vi "TEST_DialogValuesMatchINI.vi"() -> ()   [LabVIEW 2016]
uses:
  controls/ActiveDiffArgs.ctl
panel:
  out "Read from INI File":T1
  out "Settings Equal?":bool
  out "error out":errorcluster
  out "Dialog Output":T1
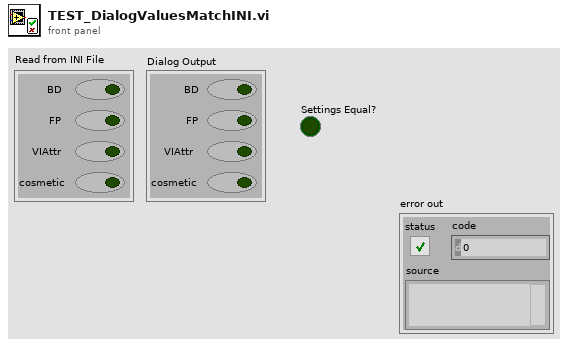
[diagram p1: front panel]
types:
  T1 = typedef "ActiveDiffArgs.ctl" = cluster{"BD":bool, "FP":bool, "VIAttr":bool, "cosmetic":bool}
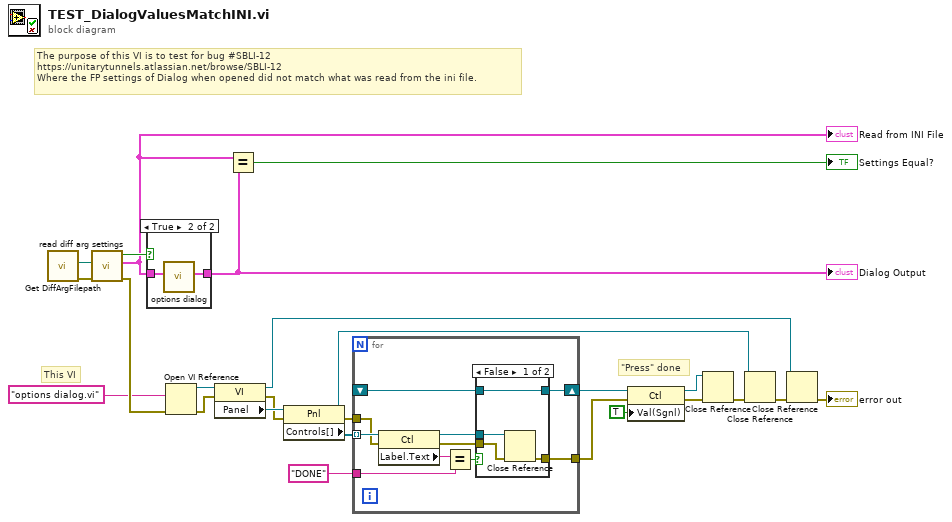
[diagram p0: block diagram]
diagram:
  # "This VI"
  # "The purpose of this VI is to test for bug #SBLI-12 \nhttps://unitarytunnels.atlassian.net/browse/SBLI-12\nWhere the FP settings of Dialog when opened did not match what was read from the ini file."
  # "\"Press\" done"
  n1 = call "Get DiffArgFilepath.vi"() -> ("error out"=w24:errorcluster, "VICompare Difftool Exe Path"=w25:path)  [unwired: 10 in]
  n2 = call "read diff arg settings.vi"("error in (no error)"=w24, "VIscc Path"=w25) -> ("error out"=w19:errorcluster, "ActiveDiffArgs"=w22:T1, "manual?"=w23:bool)  [unwired: 6 in, 1 out]
  "Read from INI File" <- w22
  n3 = case shown="True" w23 {
    tunnel: w22 -> [w26 w28]
    tunnel: [w26 w27] -> w21
    frame False {
    }
    frame True {
      n4 = call "options dialog.vi"("ActiveDiffArgs"=w28) -> ("ActiveDiffArgs out"=w27:T1)  [unwired: 10 in]
    }
  }
  "Dialog Output" <- w21
  n5 = Open VI Reference(vi path="options dialog.vi", error in (no error)=w19) -> (vi reference=w17:refnum<vi>, error out=w15:errorcluster)  [unwired: 4 in]
  n6 = property class="VI"(reference=w17, error in=w15) -> (reference out=w4:refnum<vi>, error out=w7:errorcluster, "Panel"=w14:refnum<vi>)
  n7 = Equal?(x=w22, y=w21) -> (x = y?=→"Settings Equal?":bool)
  n8 = property class="Pnl"(reference=w14, error in=w7) -> (reference out=w5:refnum<vi>, error out=w8:errorcluster, "Controls[]"=w12:refnum<vi>[])
  n9 = for {
    tunnel: w12 -> [w38] mode=indexing
    tunnel: "DONE" ("Control Name") -> [w36]
    shift-right: [w31] -> w10
    shift-left: _ -> [w32]
    tunnel: [w30] -> w9
    tunnel: w8 -> [w29]
    n10 = property class="Ctl"(reference=w38, error in=w29) -> (reference out=w35:refnum<vi>, error out=w33:errorcluster, "Label.Text"=w37:string)
    n11 = Equal?(x=w37, y=w36) -> (x = y?=w34:bool)
    n12 = case shown="False" w34 {
      tunnel: w35 -> [w42 w44]
      tunnel: w33 -> [w41 w43]
      tunnel: w32 -> [w40 _]
      tunnel: [w40 w44] -> w31
      tunnel: [w39 w43] -> w30
      frame False {
        n13 = Close Reference(reference=w42, error in (no error)=w41) -> (error out=w39:errorcluster)
      }
      frame True {
      }
    }
  }
  n14 = property class="Ctl"(reference=w10, error in=w9, "Val(Sgnl)"=TRUE) -> (reference out=w6:refnum<vi>, error out=w16:errorcluster)
  n15 = Close Reference(reference=w6, error in (no error)=w16) -> (error out=w3:errorcluster)
  n16 = Close Reference(reference=w5, error in (no error)=w3) -> (error out=w2:errorcluster)
  n17 = Close Reference(reference=w4, error in (no error)=w2) -> (error out=→"error out":errorcluster)
